vi "PC_Config (DONE).vi"(4 "Config Input":T5) -> (0 "Config Output":T8, 1 "Camera/Calibration Tab 2":refnum<vi>, 2 "New Reference Ref":refnum<vi>, 3 "Calibrate Ref":refnum<vi>)   [LabVIEW 2017]
uses:
  <vilib>/userdefined/High Color/IMAQdx.ctl
panel:
  in  "Saftey Factors":T1={"Goal Saftey Factor"=1.25, "Defender Saftey Factor"=1.8}
  in  "Puck to Step Constants":T2={"Encoder References Positions (steps)"={"X Steps"=150004.0, "Y Steps"=150000.0}, "Encoder References (mm)"={"Encoder References Start Positions (mm)"={"X Steps (Start)"=61.62, "Y Steps (Start)"=7.3}, "Encoder References End Positions (mm)"={"X Steps (End)"=171.51, "Y Steps (End)"=216.48}}, "Encoder References to Dot (steps)"={"Reference X Encoder"=229677.0, "Reference Y Encoder"=230627.0}, "Reference Dot Width (mm)"=48.8}
  in  "File Names":T3={"Grid Image Name"="..\\grid.png", "Calibration File Name"="..\\calibration.png", "Shot Image Name"="..\\table.png", "Reference Image Name"="..\\reference.png"}
  out "Puck and Defender Locations":T4
  out "Conversions":T6
  in  "Camera":T7="cam1"
  in  "Number of Erosion (Ref)":i32
  out "Theta (Best Shot)":dbl
  out "Table Walls":sgl[](array[numeric])
  in  "Puck and Player Settings":T9={"Noise Erosion"=0, "Find Circles (Min Radius)"=20.0, "Find Circles (Max Radius)"=50.0, "Cutoff Radius  "=34.0}
  out "Y Steps to Puck":dbl
  out "X Steps to Puck":dbl
  in  "Camera/Calibration Tab":T10(radio) caption="Radio Buttons"
  in  "Calibrate":bool
  in  "New Reference":bool
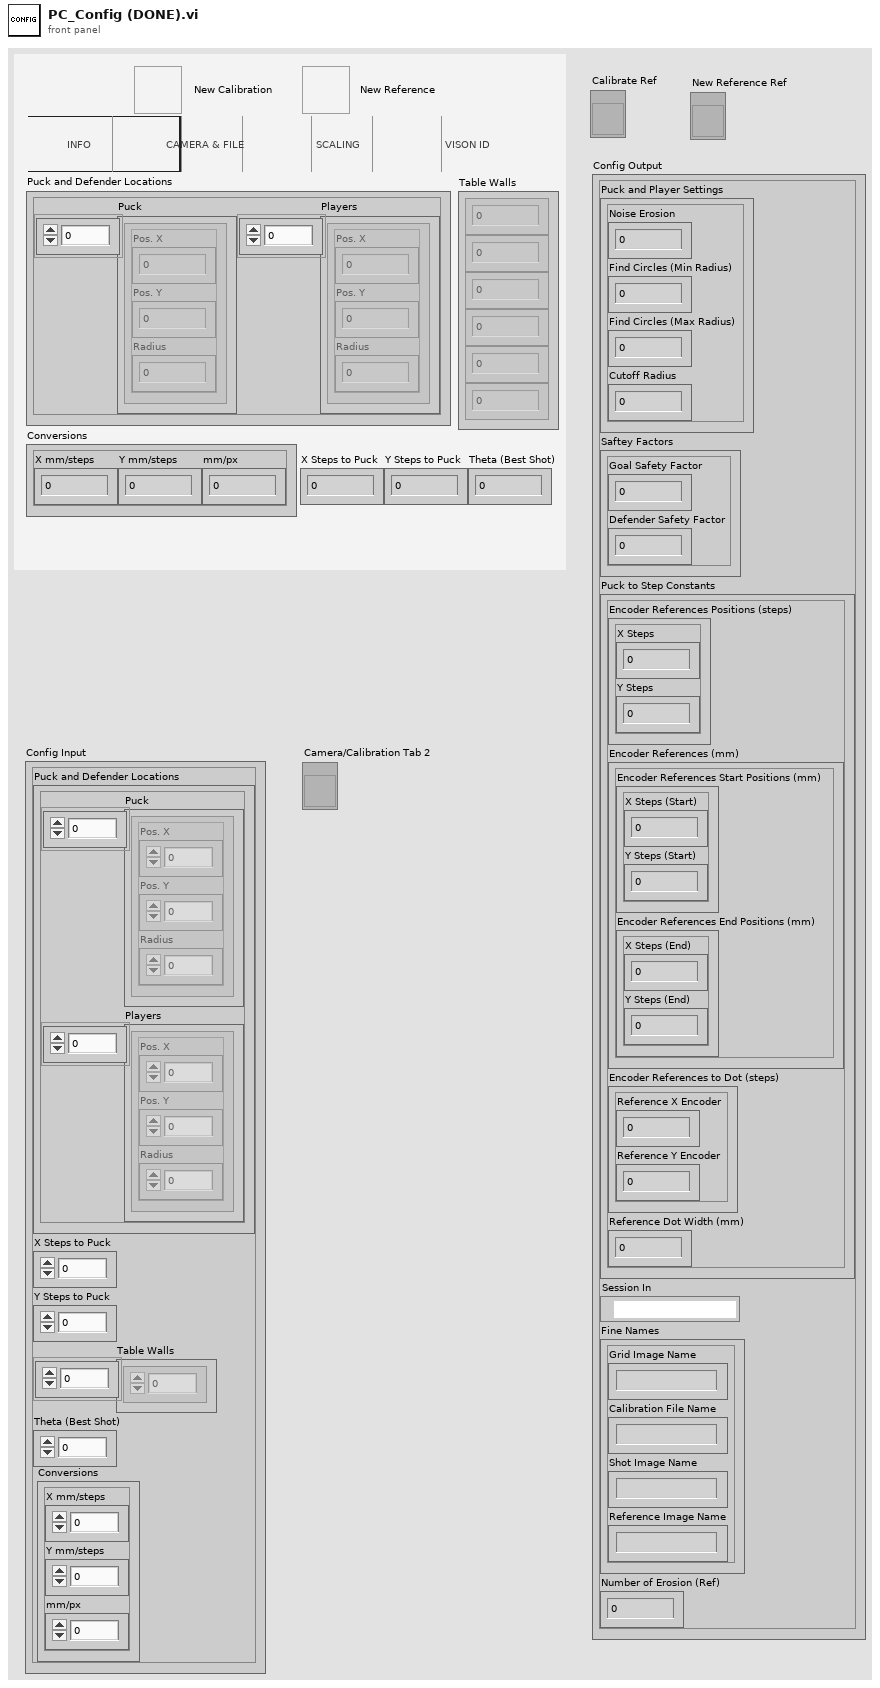
[diagram p1: front panel]
types:
  T1 = cluster{"Goal Saftey Factor":dbl, "Defender Saftey Factor":dbl}
  T2 = cluster{"Encoder References Positions (steps)":cluster{"X Steps":dbl, "Y Steps":dbl}, "Encoder References (mm)":cluster{"Encoder References Start Positions (mm)":cluster{"X Steps (Start)":dbl, "Y Steps (Start)":dbl}, "Encoder References End Positions (mm)":cluster{"X Steps (End)":dbl, "Y Steps (End)":dbl}}, "Encoder References to Dot (steps)":cluster{"Reference X Encoder":dbl, "Reference Y Encoder":dbl}, "Reference Dot Width (mm)":dbl}
  T3 = cluster{"Grid Image Name":string, "Calibration File Name":string, "Shot Image Name":string, "Reference Image Name":string}
  T4 = cluster{"Puck":cluster{"Pos. X":i32, "Pos. Y":i32, "Radius":i32}[], "Players":cluster{"Pos. X":i32, "Pos. Y":i32, "Radius":i32}[]}
  T5 = cluster{"Puck and Defender Locations":cluster{"Puck":cluster{"Pos. X":i32, "Pos. Y":i32, "Radius":i32}[], "Players":cluster{"Pos. X":i32, "Pos. Y":i32, "Radius":i32}[]}, "X Steps to Puck":dbl, "Y Steps to Puck":dbl, "Table Walls":sgl[], "Theta (Best Shot)":dbl, "Conversions":cluster{"X mm/steps":dbl, "Y mm/steps":dbl, "mm/px":dbl}}
  T6 = cluster{"X mm/steps":dbl, "Y mm/steps":dbl, "mm/px":dbl}
  T7 = typedef "IMAQdx.ctl" = refnum<k21>
  T8 = cluster{"Puck and Player Settings":cluster{"Noise Erosion":i32, "Find Circles (Min Radius)":sgl, "Find Circles (Max Radius)":sgl, "Cutoff Radius  ":sgl}, "Saftey Factors":cluster{"Goal Safety Factor":dbl, "Defender Safety Factor":dbl}, "Puck to Step Constants":cluster{"Encoder References Positions (steps)":cluster{"X Steps":dbl, "Y Steps":dbl}, "Encoder References (mm)":cluster{"Encoder References Start Positions (mm)":cluster{"X Steps (Start)":dbl, "Y Steps (Start)":dbl}, "Encoder References End Positions (mm)":cluster{"X Steps (End)":dbl, "Y Steps (End)":dbl}}, "Encoder References to Dot (steps)":cluster{"Reference X Encoder":dbl, "Reference Y Encoder":dbl}, "Reference Dot Width (mm)":dbl}, "Session In":T7, "Fine Names":cluster{"Grid Image Name":string, "Calibration File Name":string, "Shot Image Name":string, "Reference Image Name":string}, "Number of Erosion (Ref)":i32}
  T9 = cluster{"Noise Erosion":i32, "Find Circles (Min Radius)":sgl, "Find Circles (Max Radius)":sgl, "Cutoff Radius  ":sgl}
  T10 = enum32{"Camera", "Calibration", "Scaling", "Vision ID"}
  T11 = cluster{"Puck and Player Settings":cluster{"Noise Erosion":i32, "Find Circles (Min Radius)":sgl, "Find Circles (Max Radius)":sgl, "Cutoff Radius  ":sgl}, "Saftey Factors":cluster{"Goal Saftey Factor":dbl, "Defender Saftey Factor":dbl}, "Puck to Step Constants":cluster{"Encoder References Positions (steps)":cluster{"X Steps":dbl, "Y Steps":dbl}, "Encoder References (mm)":cluster{"Encoder References Start Positions (mm)":cluster{"X Steps (Start)":dbl, "Y Steps (Start)":dbl}, "Encoder References End Positions (mm)":cluster{"X Steps (End)":dbl, "Y Steps (End)":dbl}}, "Encoder References to Dot (steps)":cluster{"Reference X Encoder":dbl, "Reference Y Encoder":dbl}, "Reference Dot Width (mm)":dbl}, "Camera":T7, "File Names":cluster{"Grid Image Name":string, "Calibration File Name":string, "Shot Image Name":string, "Reference Image Name":string}, "Number of Erosion (Ref)":i32}
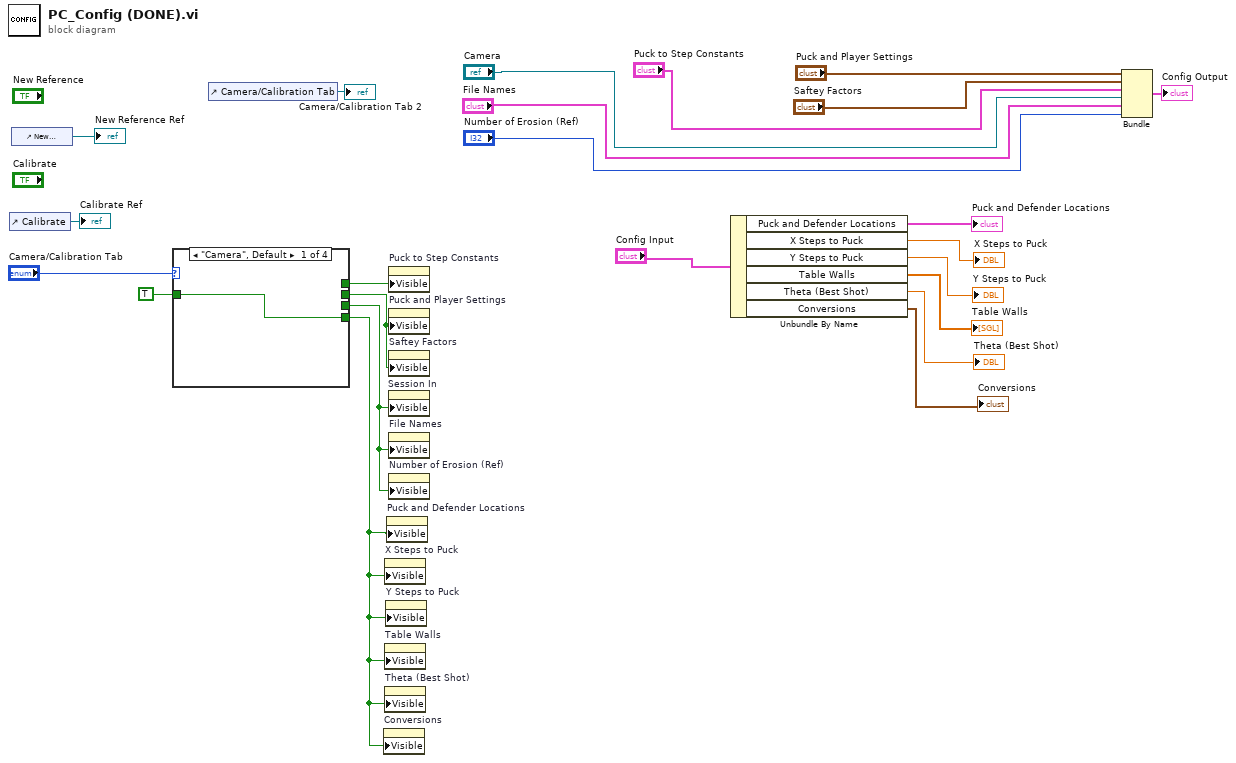
[diagram p0: block diagram]
diagram:
  n1 = control-ref of="Calibrate"() -> (→"Calibrate Ref":refnum<vi>)
  n2 = control-ref of="New Reference"() -> (→"New Reference Ref":refnum<vi>)
  n3 = case shown="\"Camera\", Default" "Camera/Calibration Tab" {
    tunnel: TRUE -> [w24 w25 w26 w27]
    tunnel: [_ _ _ w27] -> w19
    tunnel: [_ _ w26 _] -> w18
    tunnel: [_ w25 _ _] -> w17
    tunnel: [w24 _ _ _] -> w4
    frame "Camera", Default {
    }
    frame "Calibration" {
    }
    frame "Scaling" {
    }
    frame "Vision ID" {
    }
  }
  n4 = control-ref of="Camera/Calibration Tab"() -> (→"Camera/Calibration Tab 2":refnum<vi>)
  n5 = property on="Conversions" class="Clust (strict)"("Visible"=w4) -> ()  [unwired: 2 in, 2 out]
  n6 = property on="X Steps to Puck" class="DigNum (strict)"("Visible"=w4) -> ()  [unwired: 2 in, 2 out]
  n7 = property on="Table Walls" class="Arr (strict)"("Visible"=w4) -> ()  [unwired: 2 in, 2 out]
  n8 = property on="Theta (Best Shot)" class="DigNum (strict)"("Visible"=w4) -> ()  [unwired: 2 in, 2 out]
  n9 = property on="Y Steps to Puck" class="DigNum (strict)"("Visible"=w4) -> ()  [unwired: 2 in, 2 out]
  n10 = property on="Puck and Defender Locations" class="Clust (strict)"("Visible"=w4) -> ()  [unwired: 2 in, 2 out]
  n11 = property on="Puck to Step Constants" class="Clust (strict)"("Visible"=w18) -> ()  [unwired: 2 in, 2 out]
  n12 = property on="Puck and Player Settings" class="Clust (strict)"("Visible"=w19) -> ()  [unwired: 2 in, 2 out]
  n13 = property on="Saftey Factors" class="Clust (strict)"("Visible"=w19) -> ()  [unwired: 2 in, 2 out]
  n14 = property on="Session In" class="IMAQdx (strict)"("Visible"=w17) -> ()  [unwired: 2 in, 2 out]
  n15 = property on="File Names" class="Clust (strict)"("Visible"=w17) -> ()  [unwired: 2 in, 2 out]
  n16 = property on="Number of Erosion (Ref)" class="DigNum (strict)"("Visible"=w17) -> ()  [unwired: 2 in, 2 out]
  n17 = Unbundle By Name("Config Input") -> ("Puck and Defender Locations"=→"Puck and Defender Locations":T4, "X Steps to Puck"=→"X Steps to Puck":dbl, "Y Steps to Puck"=→"Y Steps to Puck":dbl, "Table Walls"=→"Table Walls":sgl[], "Theta (Best Shot)"=→"Theta (Best Shot)":dbl, "Conversions"=→"Conversions":T6)
  n18 = Bundle("Puck and Player Settings"="Puck and Player Settings", "Saftey Factors"="Saftey Factors", "Puck to Step Constants"="Puck to Step Constants", "Camera"="Camera", "File Names"="File Names", "Number of Erosion (Ref)"="Number of Erosion (Ref)") -> (→"Config Output":T11)  [unwired: 1 in]
